vi "Actor Core.vi"(8 "error in":errorcluster, 11 "SongControlsActor in":refnum<class "SongControlsActor.lvclass">) -> (0 "error out":errorcluster, 3 "Actor out":refnum<class "Actor.lvclass">)   [LabVIEW 2015, in "SongControlsActor.lvlib" / "SongControlsActor.lvclass"]
doc: "(<B>Filename</B>: Actor Framework.lvlib:Actor.lvclass:Actor Core.vi)\n\nReceives messages to the actor, reacts to them, and initiates any error handling that may shut the actor down.\n\nDescendant classes may override this VI to append parallel tasks for the actor to complete while it handles messages. Overrides use the Call Parent Method node."
uses:
  SongControlsActor.lvclass
  <vilib>/ActorFramework/Actor/Actor.lvclass
panel:
  in  "Main UI":enum32{"Main", "Debug"}(tab)
  # "Play/Pause\nSkip\nBack"
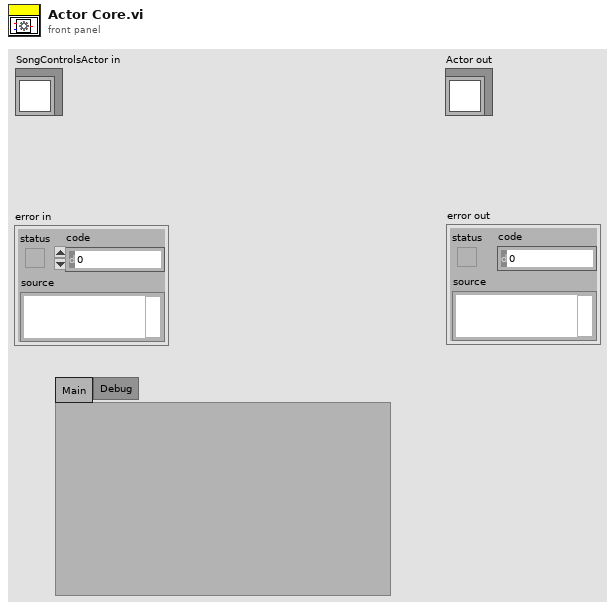
[diagram p1: front panel]
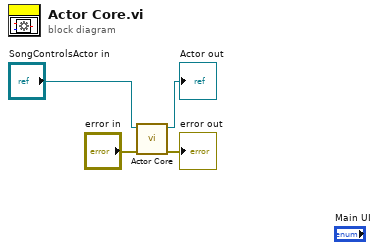
[diagram p0: block diagram]
diagram:
  n1 = call-parent "Actor Core.vi"("error in"="error in", "Actor in"="SongControlsActor in") -> ("error out"=→"error out":errorcluster, "Actor out"=→"Actor out":refnum<class "Actor.lvclass">)  [unwired: 8 in]
